vi "Write Run Block.vi"(8 "error in (no error)":errorcluster, 10 "Run block":refnum<class "Run Block.lvclass">, 11 "Monkey in":refnum<class "Monkey.lvclass">=refnum) -> (0 "error out":errorcluster, 3 "Monkey out":refnum<class "Monkey.lvclass">)   [LabVIEW 2020, in "CIRCUS_uServices.lvlib" / "Monkey.lvlib" / "Monkey.lvclass"]
uses:
  Monkey.lvclass
  Monkey.lvclass/Monkey.ctl
  Run Utilities/Run Block/Run Block.lvclass
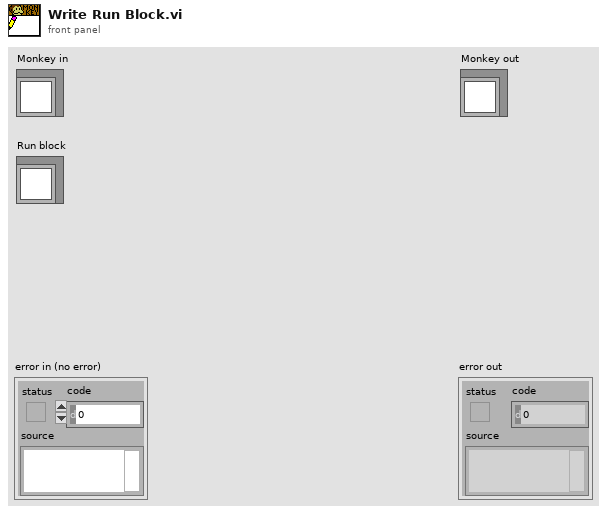
[diagram p1: front panel]
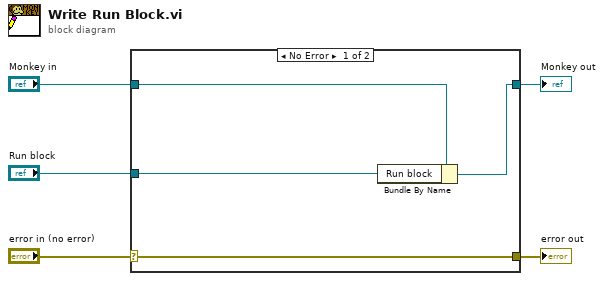
[diagram p0: block diagram]
diagram:
  n1 = case shown="No Error" "error in (no error)" {
    selector: "error in (no error)" -> [w9 w10]
    tunnel: [w9 w10] -> w4
    tunnel: [w7 w11] -> w2
    tunnel: "Monkey in" -> [w8 w11]
    tunnel: "Run block" -> [w6 _]
    frame No Error {
      n2 = Bundle By Name(cluster=w8, "Run block"=w6) -> (w7:refnum<class "Monkey.lvclass">)
    }
    frame Error {
    }
  }
  "error out" <- w4
  "Monkey out" <- w2
